vi "Initialize.vi"(8 "error in (no error)":errorcluster, 10 "Baud Rate (115200)":u32=115200, 11 "VISA resource name":refnum<visa-resource-name>) -> (0 "error out":errorcluster, 3 "VISA resource name out":refnum<visa-resource-name>)   [LabVIEW 2018, in "Zaber A Series.lvlib"]
doc: "Establishes communication with a Zaber device and clears the serial buffer. Call this VI before calling other instrument driver VIs for this instrument. You need to call the Initialize VI only once at the beginning of an application, or again after using the Close VI. \n\nNote: \nThe default baud rate for the ASCII protocol is 115200, but the devices can be adjusted to use different baud rates in which case you should adjust the baud rate indicator."
uses:
  Zaber A Series.lvlib
  <vilib>/Instr/_visa.llb/VISA Configure Serial Port (Instr).vi
panel:
  # "(c) 2017-2020 Zaber Technologies.  ALL RIGHTS RESERVED."
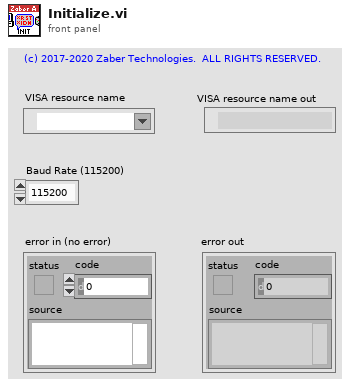
[diagram p1: front panel]
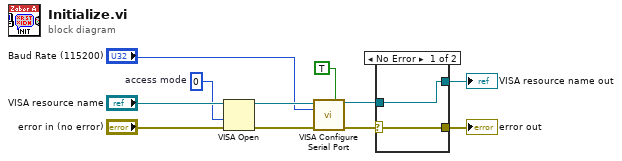
[diagram p0: block diagram]
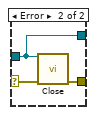
[diagram p2: hidden frame]
diagram:
  w9 = u32 0  # access mode
  n1 = VISA Open(access mode=w9, error in (no error)="error in (no error)", VISA resource name="VISA resource name") -> (VISA resource name=w3:refnum<visa-resource-name>, error out=w4:errorcluster)  [unwired: 2 in]
  n2 = call-poly "VISA Configure Serial Port"("VISA resource name"=w3, "Enable Termination\nChar (T)"=TRUE ("Enable Termination\nChar (T)"), "baud rate (9600)"="Baud Rate (115200)", "error in (no error)"=w4) -> ("VISA resource name out"=w6:refnum<visa-resource-name>, "error out"=w5:errorcluster)  [unwired: 10 in]
  n3 = case shown="No Error" w5 {
    selector: w5 -> [w12 w15]
    tunnel: w6 -> [w13 w14]
    tunnel: [w13 w14] -> w8
    tunnel: [w12 w16] -> w7
    frame No Error {
    }
    frame Error {
      n4 = call "Close.vi"("error in (no error)"=w15, "VISA resource name"=w14) -> ("error out"=w16:errorcluster)  [unwired: 9 in]
    }
  }
  "VISA resource name out" <- w8
  "error out" <- w7
